vi "fgv_DS1202_data.vi"(7 "cmd":T1, 11 "wfm":waveform(dbl)(graph)={"t0"=timestamp(0 s since 1904-01-01), "dt"=2.0000000000000002e-07, "Y"=array[1202 elements]}) -> (3 "wfm 2":waveform(dbl))   [LabVIEW 2021]
uses:
  ctrl/rw.ctl
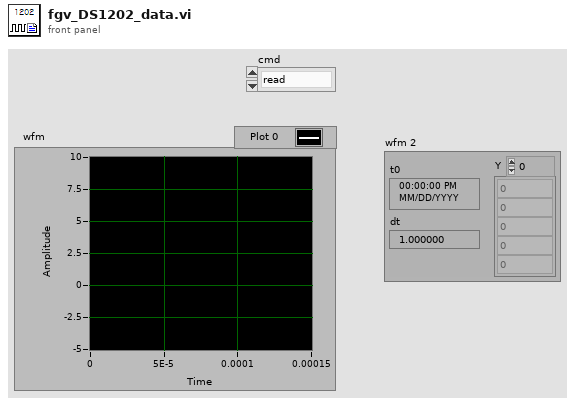
[diagram p1: front panel]
types:
  T1 = typedef "rw.ctl" = enum16{"read", "write"}
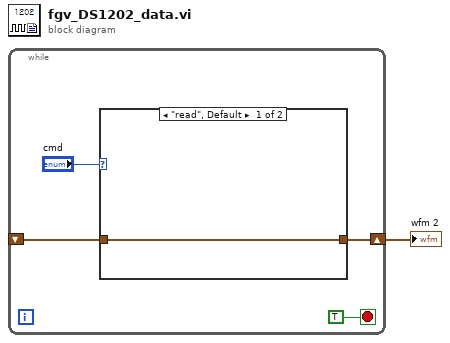
[diagram p0: block diagram]
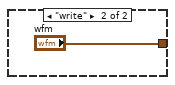
[diagram p2: hidden frame]
diagram:
  n1 = while {
    shift-right: [w3] -> w1
    shift-left: _ -> [w2]
    stop <- TRUE stop-if-true
    n2 = case shown="\"read\", Default" "cmd" {
      tunnel: [w6 "wfm"] -> w3
      tunnel: w2 -> [w6 _]
      frame "read", Default {
      }
      frame "write" {
      }
    }
  }
  "wfm 2" <- w1
